vi "Setup.vi"() -> (3 "Data":map{string, variant[]}(c390))   [LabVIEW 2023]
uses:
  LV-Argparse/LV Argument Parser/Argument Definition.ctl
  LV-Argparse/LV Argument Parser/LV Argument Parser.lvclass/LV Argument Parser.ctl
  0769afa5-ade5-446d-90ea-3acaa0259a06.vi
  LV-Argparse/LV Argument Parser/Read Data.vi
  LV-Argparse/LV Argument Parser/Parse.vi
  LV-Argparse/LV Argument Parser/Obtain.vi
  LV-Argparse/LV Argument Parser/Get.vi
  LV-Argparse/LV Argument Parser/LV Argument Parser.lvclass
  LV-Argparse/LV ArgParse.lvlib
panel:
  out "Output":string
  in  "Args":string="-n 1 -n 2 --config C:\\bla.ini \"Blablabla\""
  out "data":u32[](array[numeric])
  out "error out":errorcluster
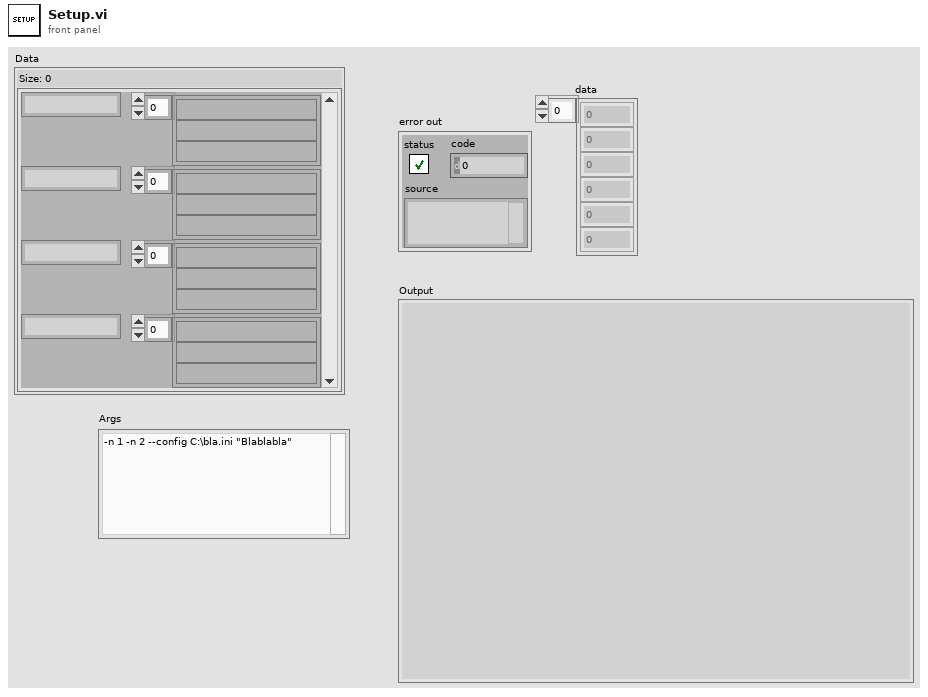
[diagram p1: front panel]
types:
  T1 = typedef "LV ArgParse.lvlib/LV Argument Parser.lvclass/Argument Definition.ctl" = cluster{"Name":string, "short (positional)":string, "long (positional)":string, "action":enum16{"store", "store-const", "store-false", "store-true", "append", "append-const", "count", "help", "version"}, "choices":string[], "const":string, "default":string, "dest (=name)":string, "help":string, "Number":i32, "Required":bool, "Type":enum16{"String", "Int", "Uint", "Float", "Bool", "Date", "Path"}}
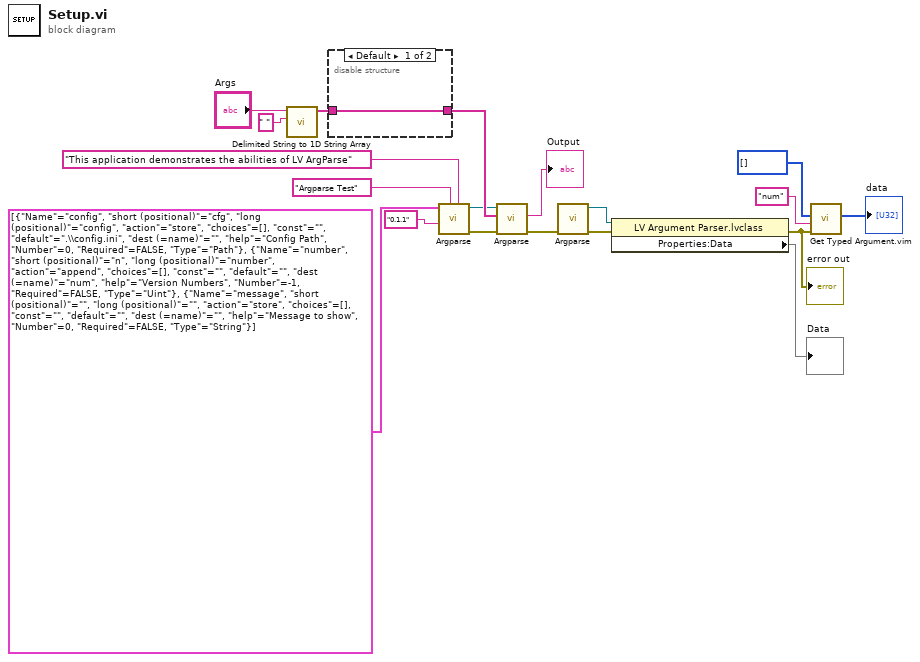
[diagram p0: block diagram]
diagram:
  n1 = call <vilib>:"Delimited String to 1D String Array.vi"("delimiter"=" ", "delimited string"="Args") -> ("string array"=w15:string[])  [unwired: 9 in]
  n2 = disable-structure shown="Default" {
    disable-tunnel: [w20 _] -> w7
    disable-tunnel: w15 -> [w20 _]
    frame condition #0 (active) {
    }
    frame condition #1 {
    }
  }
  n3 = call-poly "Argparse.vi"("Description"="This application demonstrates the abilities of LV ArgParse", "Name"="Argparse Test", "Version"="0.1.1", "Arguments"=T1[] [{"Name"="config", "short (positional)"="cfg", "long (positional)"="config", "action"=enum."store", "choices"=[], "const"="", "default"=".\\config.ini", "dest (=name)"="", "help"="Config Path", "Number"=0, "Required"=FALSE, "Type"=enum."Path"}, {"Name"="number", "short (positional)"="n", "long (positional)"="number", "action"=enum."append", "choices"=[], "const"="", "default"="", "dest (=name)"="num", "help"="Version Numbers", "Number"=-1, "Required"=FALSE, "Type"=enum."Uint"}, {"Name"="message", "short (positional)"="", "long (positional)"="", "action"=enum."store", "choices"=[], "const"="", "default"="", "dest (=name)"="", "help"="Message to show", "Number"=0, "Required"=FALSE, "Type"=enum."String"}]) -> ("error out"=w14:errorcluster, "LV Argument Parser out"=w5:refnum<class "LV Argument Parser.lvclass">)  [unwired: 6 in]
  n4 = call-poly "Argparse.vi"("error in (no error)"=w14, "Arguments (From Args)"=w7, "LV Argument Parser in (Global)"=w5) -> ("error out"=w13:errorcluster, "Output"=→"Output":string)  [unwired: 6 in, 1 out]
  n5 = call-poly "Argparse.vi"("error in (no error)"=w13) -> ("error out"=w4:errorcluster, "LV Argument Parser out"=w9:refnum<class "LV Argument Parser.lvclass">)  [unwired: 9 in]
  n6 = property class="LV Argument Parser.lvclass"(reference=w9, error in=w4) -> (error out=w1:errorcluster, "Properties:Data"=→"Data":map{string, variant[]})  [unwired: 1 out]
  "error out" <- w1
  n7 = call "Get Typed Argument.vim"("error in (no error)"=w1, "Name"="num", "Type / Default"=u32[] []) -> ("data"=→"data":u32[])  [unwired: 6 in, 2 out]
